vi "Get Parent Window Bounds.vi"(8 "error in (no error)":errorcluster, 11 "Parent Hwnd":i32) -> (0 "error out":errorcluster, 2 "Bounds":T1, 3 "Hwnd Out":i32)   [LabVIEW 2016, in "LV MDI.lvclass"]
doc: "Retrieves the dimensions of the bounding rectangle of the specified parent window."
uses:
  LV MDI.lvclass
  protected/Offset.ctl
  user32.dll
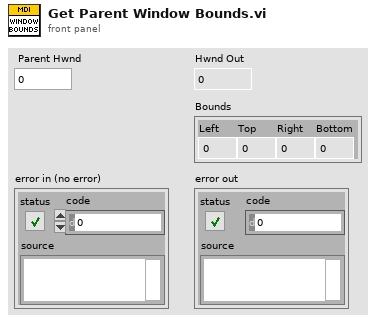
[diagram p1: front panel]
types:
  T1 = typedef "LV MDI.lvclass/Offset.ctl" = cluster{"Left":i32, "Top":i32, "Right":i32, "Bottom":i32}
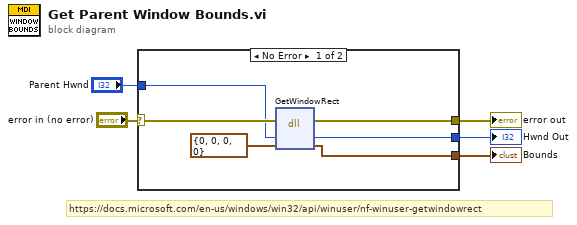
[diagram p0: block diagram]
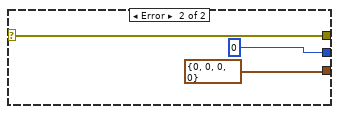
[diagram p2: hidden frame]
diagram:
  # "https://docs.microsoft.com/en-us/windows/win32/api/winuser/nf-winuser-getwindowrect"
  n1 = case shown="No Error" "error in (no error)" {
    selector: "error in (no error)" -> [w7 w14]
    tunnel: [w11 0 ("Hwnd")] -> w5
    tunnel: [w10 T1 {"Left"=0, "Top"=0, "Right"=0, "Bottom"=0} ("lpRect")] -> w4
    tunnel: [w8 w14] -> w3
    tunnel: "Parent Hwnd" -> [w6 _]
    frame No Error {
      n2 = dll-call lib="user32.dll" fn="GetWindowRect"(error in=w7, "Hwnd"=w6, "lpRect"=T1 {"Left"=0, "Top"=0, "Right"=0, "Bottom"=0} ("Offset Rect")) -> (error out=w8:errorcluster, "Hwnd"=w11:i32, "lpRect"=w10:T1)  [unwired: 3 in, 1 out]
    }
    frame Error {
    }
  }
  "Hwnd Out" <- w5
  "Bounds" <- w4
  "error out" <- w3
